vi "Periodic Tasks.vi"(8 "error in":errorcluster) -> ()   [LabVIEW 2023]
doc: "This VI runs in parallel to other tasks. It can contain as many user-defined periodic loops as you need. These can carry out PID or other sorts of timed response."
uses:
  <vilib>/Rock Robotics/WPI/DriverStation/WPI_DriverStationAllianceInfo.ctl
  GeneralPurpose/AllianceColorGlobal.vi
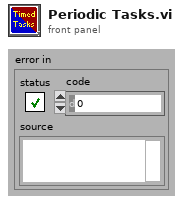
[diagram p1: front panel]
types:
  T1 = typedef "WPI_DriverStationAllianceInfo.ctl" = enum16{"Red", "Blue", "Invalid"}
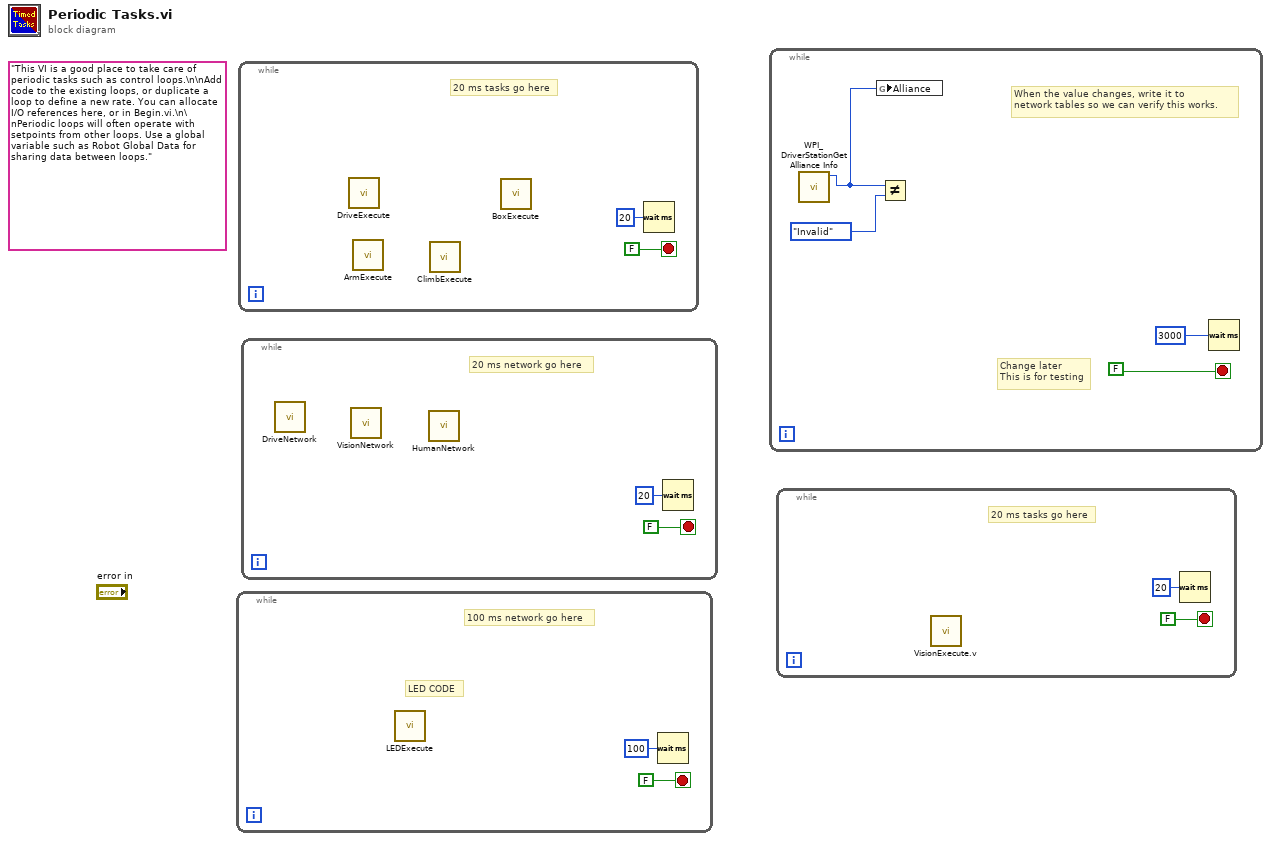
[diagram p0: block diagram]
diagram:
  (unwired) "This VI is a good place to take care of periodic tasks such as control loops.\n\nAdd code to the existing loops, or duplicate a loop to define a new rate. You can allocate I/O references here, or in Begin.vi.\n\nPeriodic loops will often operate with setpoints from other loops. Use a global variable such as Robot Global Data for sharing data between loops."
  n1 = while {
    stop <- FALSE stop-if-true
    # "LED CODE"
    # "100 ms network go here"
    n2 = call "LEDExecute.vi"() -> ()  [unwired: 12 in]
    n3 = Wait (ms)(milliseconds to wait=u32 100) -> ()  [unwired: 1 out]
  }
  n4 = while {
    stop <- FALSE stop-if-true
    # "20 ms tasks go here"
    n5 = call "DriveExecute.vi"() -> ()  [unwired: 11 in, 1 out]
    n6 = call "ArmExecute.vi"() -> ()  [unwired: 11 in, 1 out]
    n7 = call "ClimbExecute.vi"() -> ()  [unwired: 11 in, 1 out]
    n8 = call "BoxExecute.vi"() -> ()  [unwired: 11 in, 1 out]
    n9 = Wait (ms)(milliseconds to wait=u32 20) -> ()  [unwired: 1 out]
  }
  n10 = while {
    stop <- FALSE stop-if-true
    # "20 ms network go here"
    n11 = call "DriveNetwork.vi"() -> ()  [unwired: 11 in, 1 out]
    n12 = call "VisionNetwork.vi"() -> ()  [unwired: 11 in, 1 out]
    n13 = call "HumanNetwork.vi"() -> ()  [unwired: 11 in, 1 out]
    n14 = Wait (ms)(milliseconds to wait=u32 20) -> ()  [unwired: 1 out]
  }
  n15 = while {
    stop <- FALSE stop-if-true
    # "When the value changes, write it to \nnetwork tables so we can verify this works."
    # "Change later\nThis is for testing"
    n16 = call <vilib>:"WPI_DriverStationGet Alliance Info.vi"() -> ("Alliance"=w7:T1)  [unwired: 6 in, 5 out]
    n17 = global write "AllianceColorGlobal.vi" "Alliance"(w7) -> ()
    n18 = Not Equal?(x=w7, y=WPI_DriverStationAllianceInfo."Invalid") -> ()  [unwired: 1 out]
    n19 = Wait (ms)(milliseconds to wait=u32 3000) -> ()  [unwired: 1 out]
  }
  n20 = while {
    stop <- FALSE stop-if-true
    # "20 ms tasks go here"
    n21 = call "VisionExecute.v.vi"() -> ()  [unwired: 12 in]
    n22 = Wait (ms)(milliseconds to wait=u32 20) -> ()  [unwired: 1 out]
  }
